vi "example_cmd.vi"() -> ()   [LabVIEW 2015]
uses:
  dotnet_system_exec/dotnet_system_exec.lvclass
panel:
  in  "working directory":path=path "c:/"
  out "StdErr":string
  out "StdOut":string
  in  "Send":bool
  in  "Cmd In (can include multiple lines)":string="dir"
  in  "Stop":bool
  # "This examples launches the cmd.exe process and allows you to send strings via stdin, while asynchronously listening to stdout and stderr  \n\nCalling \"exit\" in CmdIn will stop the cmd.exe instance and stop this VI. You can leverage this by adding a final exit line after the command(s)\nyou wish to send to have this VI auto-terminate upon completion."
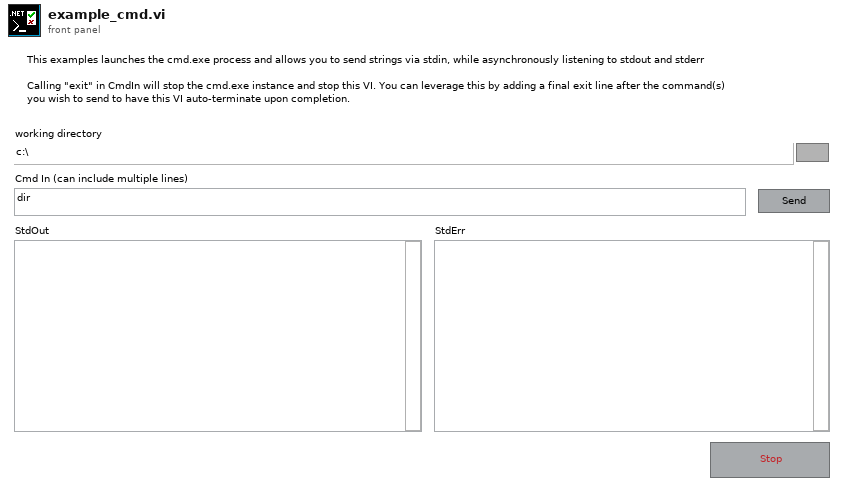
[diagram p1: front panel]
types:
  T1 = cluster{"stdout event":refnum<user-event>, "stderr event":refnum<user-event>, "process_exit event":refnum<user-event>}
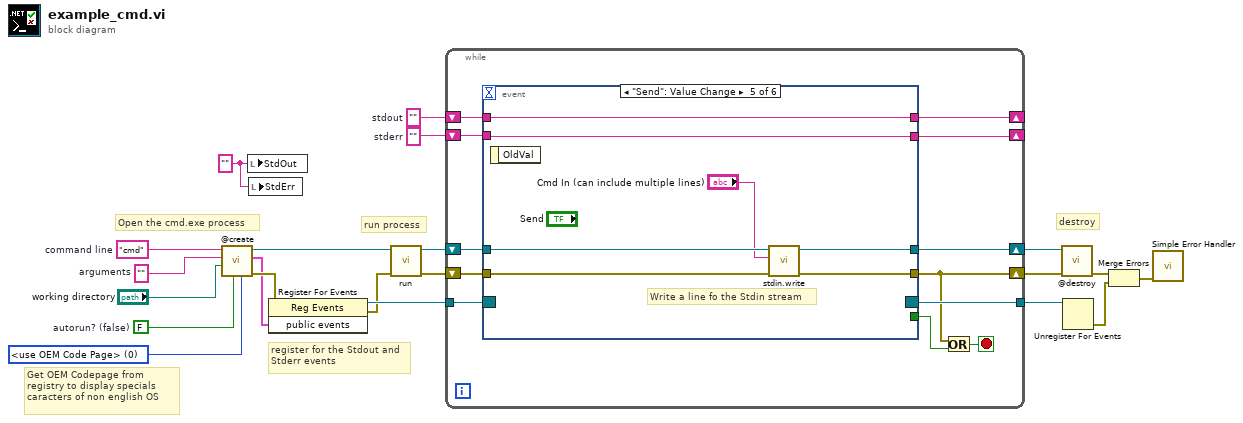
[diagram p0: block diagram]
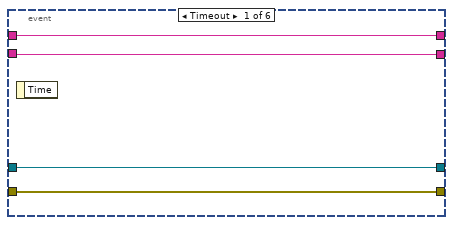
[diagram p2: hidden frame]
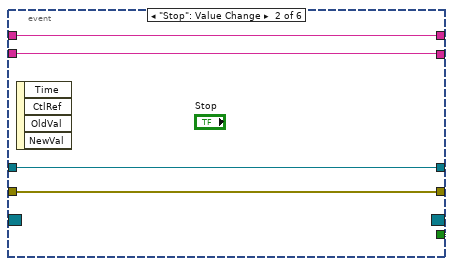
[diagram p3: hidden frame]
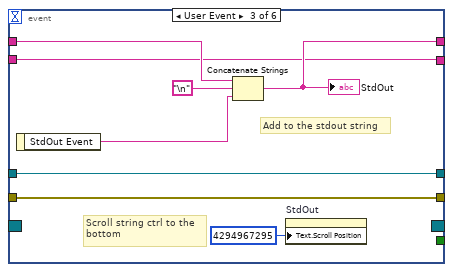
[diagram p4: hidden frame]
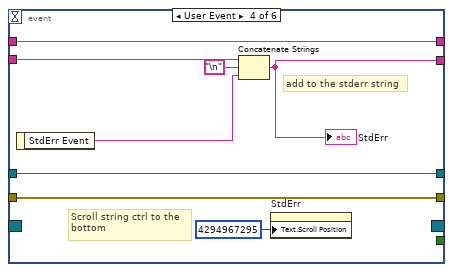
[diagram p5: hidden frame]
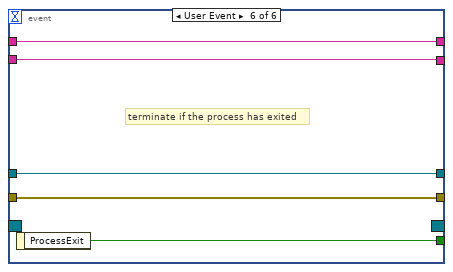
[diagram p6: hidden frame]
diagram:
  w1 = 0 items=["<do not specify>"=-1, "<use OEM Code Page>"=0, "IBM037 - IBM EBCDIC US-Canada"=37, "IBM437 - OEM United States"=437, "IBM500 - IBM EBCDIC International"=500, "ASMO-708 - Arabic (ASMO 708)"=708, "709 - Arabic (ASMO-449+, BCON V4)"=709, "710 - Arabic - Transparent Arabic"=710, "DOS-720 - Arabic (Transparent ASMO); Arabic (DOS)"=720, "ibm737 - OEM Greek (formerly 437G); Greek (DOS)"=737, "ibm775 - OEM Baltic; Baltic (DOS)"=775, "ibm850 - OEM Multilingual Latin 1; Western European (DOS)"=850, "ibm852 - OEM Latin 2; Central European (DOS)"=852, "IBM855 - OEM Cyrillic (primarily Russian)"=855, "ibm857 - OEM Turkish; Turkish (DOS)"=857, "IBM00858 - OEM Multilingual Latin 1 + Euro symbol"=858, "IBM860 - OEM Portuguese; Portuguese (DOS)"=860, "ibm861 - OEM Icelandic; Icelandic (DOS)"=861, "DOS-862 - OEM Hebrew; Hebrew (DOS)"=862, "IBM863 - OEM French Canadian; French Canadian (DOS)"=863, "IBM864 - OEM Arabic; Arabic (864)"=864, "IBM865 - OEM Nordic; Nordic (DOS)"=865, "cp866 - OEM Russian; Cyrillic (DOS)"=866, "ibm869 - OEM Modern Greek; Greek, Modern (DOS)"=869, "IBM870 - IBM EBCDIC Multilingual/ROECE (Latin 2); IBM EBCDIC Multilingual Latin 2"=870, "windows-874 - Thai (Windows)"=874, "cp875 - IBM EBCDIC Greek Modern"=875, "shift_jis - ANSI/OEM Japanese; Japanese (Shift-JIS)"=932, "gb2312 - ANSI/OEM Simplified Chinese (PRC, Singapore); Chinese Simplified (GB2312)"=936, "ks_c_5601-1987 - ANSI/OEM Korean (Unified Hangul Code)"=949, "big5 - ANSI/OEM Traditional Chinese (Taiwan; Hong Kong SAR, PRC); Chinese Traditional (Big5)"=950, "IBM1026 - IBM EBCDIC Turkish (Latin 5)"=1026, "IBM01047 - IBM EBCDIC Latin 1/Open System"=1047, "IBM01140 - IBM EBCDIC US-Canada (037 + Euro symbol); IBM EBCDIC (US-Canada-Euro)"=1140, "IBM01141 - IBM EBCDIC Germany (20273 + Euro symbol); IBM EBCDIC (Germany-Euro)"=1141, "IBM01142 - IBM EBCDIC Denmark-Norway (20277 + Euro symbol); IBM EBCDIC (Denmark-Norway-Euro)"=1142, "IBM01143 - IBM EBCDIC Finland-Sweden (20278 + Euro symbol); IBM EBCDIC (Finland-Sweden-Euro)"=1143, "IBM01144 - IBM EBCDIC Italy (20280 + Euro symbol); IBM EBCDIC (Italy-Euro)"=1144, "IBM01145 - IBM EBCDIC Latin America-Spain (20284 + Euro symbol); IBM EBCDIC (Spain-Euro)"=1145, "IBM01146 - IBM EBCDIC United Kingdom (20285 + Euro symbol); IBM EBCDIC (UK-Euro)"=1146, "IBM01147 - IBM EBCDIC France (20297 + Euro symbol); IBM EBCDIC (France-Euro)"=1147, "IBM01148 - IBM EBCDIC International (500 + Euro symbol); IBM EBCDIC (International-Euro)"=1148, "IBM01149 - IBM EBCDIC Icelandic (20871 + Euro symbol); IBM EBCDIC (Icelandic-Euro)"=1149, "utf-16 - Unicode UTF-16, little endian byte order (BMP of ISO 10646); available only to managed applications"=1200, "unicodeFFFE - Unicode UTF-16, big endian byte order; available only to managed applications"=1201, "windows-1250 - ANSI Central European; Central European (Windows)"=1250, "windows-1251 - ANSI Cyrillic; Cyrillic (Windows)"=1251, "windows-1252 - ANSI Latin 1; Western European (Windows)"=1252, "windows-1253 - ANSI Greek; Greek (Windows)"=1253, "windows-1254 - ANSI Turkish; Turkish (Windows)"=1254, "windows-1255 - ANSI Hebrew; Hebrew (Windows)"=1255, "windows-1256 - ANSI Arabic; Arabic (Windows)"=1256, "windows-1257 - ANSI Baltic; Baltic (Windows)"=1257, "windows-1258 - ANSI/OEM Vietnamese; Vietnamese (Windows)"=1258, "Johab - Korean (Johab)"=1361, "macintosh - MAC Roman; Western European (Mac)"=10000, "x-mac-japanese - Japanese (Mac)"=10001, "x-mac-chinesetrad - MAC Traditional Chinese (Big5); Chinese Traditional (Mac)"=10002, "x-mac-korean - Korean (Mac)"=10003, "x-mac-arabic - Arabic (Mac)"=10004, "x-mac-hebrew - Hebrew (Mac)"=10005, "x-mac-greek - Greek (Mac)"=10006, "x-mac-cyrillic - Cyrillic (Mac)"=10007, "x-mac-chinesesimp - MAC Simplified Chinese (GB 2312); Chinese Simplified (Mac)"=10008, "x-mac-romanian - Romanian (Mac)"=10010, "x-mac-ukrainian - Ukrainian (Mac)"=10017, "x-mac-thai - Thai (Mac)"=10021, "x-mac-ce - MAC Latin 2; Central European (Mac)"=10029, "x-mac-icelandic - Icelandic (Mac)"=10079, "x-mac-turkish - Turkish (Mac)"=10081, "x-mac-croatian - Croatian (Mac)"=10082, "utf-32 - Unicode UTF-32, little endian byte order; available only to managed applications"=12000, "utf-32BE - Unicode UTF-32, big endian byte order; available only to managed applications"=12001, "x-Chinese_CNS - CNS Taiwan; Chinese Traditional (CNS)"=20000, "x-cp20001 - TCA Taiwan"=20001, "x_Chinese-Eten - Eten Taiwan; Chinese Traditional (Eten)"=20002, "x-cp20003 - IBM5550 Taiwan"=20003, "x-cp20004 - TeleText Taiwan"=20004, "x-cp20005 - Wang Taiwan"=20005, "x-IA5 - IA5 (IRV International Alphabet No. 5, 7-bit); Western European (IA5)"=20105, "x-IA5-German - IA5 German (7-bit)"=20106, "x-IA5-Swedish - IA5 Swedish (7-bit)"=20107, "x-IA5-Norwegian - IA5 Norwegian (7-bit)"=20108, "us-ascii - US-ASCII (7-bit)"=20127, "x-cp20261 - T.61"=20261, "x-cp20269 - ISO 6937 Non-Spacing Accent"=20269, "IBM273 - IBM EBCDIC Germany"=20273, "IBM277 - IBM EBCDIC Denmark-Norway"=20277, "IBM278 - IBM EBCDIC Finland-Sweden"=20278, "IBM280 - IBM EBCDIC Italy"=20280, "IBM284 - IBM EBCDIC Latin America-Spain"=20284, "IBM285 - IBM EBCDIC United Kingdom"=20285, "IBM290 - IBM EBCDIC Japanese Katakana Extended"=20290, "IBM297 - IBM EBCDIC France"=20297, "IBM420 - IBM EBCDIC Arabic"=20420, "IBM423 - IBM EBCDIC Greek"=20423, "IBM424 - IBM EBCDIC Hebrew"=20424, "x-EBCDIC-KoreanExtended - IBM EBCDIC Korean Extended"=20833, "IBM-Thai - IBM EBCDIC Thai"=20838, "koi8-r - Russian (KOI8-R); Cyrillic (KOI8-R)"=20866, "IBM871 - IBM EBCDIC Icelandic"=20871, "IBM880 - IBM EBCDIC Cyrillic Russian"=20880, "IBM905 - IBM EBCDIC Turkish"=20905, "IBM00924 - IBM EBCDIC Latin 1/Open System (1047 + Euro symbol)"=20924, "EUC-JP - Japanese (JIS 0208-1990 and 0212-1990)"=20932, "x-cp20936 - Simplified Chinese (GB2312); Chinese Simplified (GB2312-80)"=20936, "x-cp20949 - Korean Wansung"=20949, "cp1025 - IBM EBCDIC Cyrillic Serbian-Bulgarian"=21025, "21027 - (deprecated)"=21027, "koi8-u - Ukrainian (KOI8-U); Cyrillic (KOI8-U)"=21866, "iso-8859-1 - ISO 8859-1 Latin 1; Western European (ISO)"=28591, "iso-8859-2 - ISO 8859-2 Central European; Central European (ISO)"=28592, "iso-8859-3 - ISO 8859-3 Latin 3"=28593, "iso-8859-4 - ISO 8859-4 Baltic"=28594, "iso-8859-5 - ISO 8859-5 Cyrillic"=28595, "iso-8859-6 - ISO 8859-6 Arabic"=28596, "iso-8859-7 - ISO 8859-7 Greek"=28597, "iso-8859-8 - ISO 8859-8 Hebrew; Hebrew (ISO-Visual)"=28598, "iso-8859-9 - ISO 8859-9 Turkish"=28599, "iso-8859-13 - ISO 8859-13 Estonian"=28603, "iso-8859-15 - ISO 8859-15 Latin 9"=28605, "x-Europa - Europa 3"=29001, "iso-8859-8-i - ISO 8859-8 Hebrew; Hebrew (ISO-Logical)"=38598, "iso-2022-jp - ISO 2022 Japanese with no halfwidth Katakana; Japanese (JIS)"=50220, "csISO2022JP - ISO 2022 Japanese with halfwidth Katakana; Japanese (JIS-Allow 1 byte Kana)"=50221, "iso-2022-jp - ISO 2022 Japanese JIS X 0201-1989; Japanese (JIS-Allow 1 byte Kana - SO/SI)"=50222, "iso-2022-kr - ISO 2022 Korean"=50225, "x-cp50227 - ISO 2022 Simplified Chinese; Chinese Simplified (ISO 2022)"=50227, "50229 - ISO 2022 Traditional Chinese"=50229, "50930 - EBCDIC Japanese (Katakana) Extended"=50930, "50931 - EBCDIC US-Canada and Japanese"=50931, "50933 - EBCDIC Korean Extended and Korean"=50933, "50935 - EBCDIC Simplified Chinese Extended and Simplified Chinese"=50935, "50936 - EBCDIC Simplified Chinese"=50936, "50937 - EBCDIC US-Canada and Traditional Chinese"=50937, "50939 - EBCDIC Japanese (Latin) Extended and Japanese"=50939, "euc-jp - EUC Japanese"=51932, "EUC-CN - EUC Simplified Chinese; Chinese Simplified (EUC)"=51936, "euc-kr - EUC Korean"=51949, "51950 - EUC Traditional Chinese"=51950, "hz-gb-2312 - HZ-GB2312 Simplified Chinese; Chinese Simplified (HZ)"=52936, "GB18030 - Windows XP and later: GB18030 Simplified Chinese (4 byte); Chinese Simplified (GB18030)"=54936, "x-iscii-de - ISCII Devanagari"=57002, "x-iscii-be - ISCII Bangla"=57003, "x-iscii-ta - ISCII Tamil"=57004, "x-iscii-te - ISCII Telugu"=57005, "x-iscii-as - ISCII Assamese"=57006, "x-iscii-or - ISCII Odia"=57007, "x-iscii-ka - ISCII Kannada"=57008, "x-iscii-ma - ISCII Malayalam"=57009, "x-iscii-gu - ISCII Gujarati"=57010, "x-iscii-pa - ISCII Punjabi"=57011, "utf-7 - Unicode (UTF-7)"=65000, "utf-8 - Unicode (UTF-8)"=65001] ("CodePage (<do not specify>)")
  w2 = FALSE  # autorun? (false)
  w3 = "" ("Process File Name")
  w5 = ""  # stderr
  w10 = ""  # arguments
  w11 = ""  # stdout
  w12 = "cmd"  # command line
  # "Get OEM Codepage from registry to display specials caracters of non english OS"
  # "destroy"
  # "register for the Stdout and\nStderr events"
  # "run process"
  # "Open the cmd.exe process"
  n1 = call "@create.vi"("CodePage (<do not specify>)"=w1, "autorun? (false)"=w2, "working directory (c:\\)"="working directory", "arguments (\"\")"=w10, "command line (cmd.exe)"=w12) -> ("error out"=w8:errorcluster, "public events"=w6:T1, "dotnet_system_exec out"=w19:refnum<class "dotnet_system_exec.lvclass">)  [unwired: 4 in]
  n2 = local write "StdOut"(w3) -> ()
  n3 = local write "StdErr"(w3) -> ()
  n4 = register-events(error in=w8, w6) -> (reference out=w18:refnum<event-registration>, error out=w7:errorcluster)  [unwired: 1 in]
  n5 = call "run.vi"("error in (no error)"=w7, "dotnet_system_exec in"=w19) -> ("error out"=w9:errorcluster, "dotnet_system_exec out"=w21:refnum<class "dotnet_system_exec.lvclass">)  [unwired: 8 in]
  n6 = while {
    shift-right: [w33] -> w20
    shift-left: w21 -> [w32]
    shift-right: [w23] -> w16
    shift-left: w9 -> [w31]
    tunnel: w18 -> [w30]
    tunnel: [w29] -> w17
    shift-right: [w27] -> _
    shift-left: w11 -> [w28]
    shift-right: [w25] -> _
    shift-left: w5 -> [w26]
    stop <- w22 stop-if-true
    n7 = event shown="[4] \"Send\": Value Change" {
      selector: w30 -> [_ _ _ _ _ _]
      dyn-events: [_ _ _ _ _ _] -> w29
      timeout: _ -> [_ _ _ _ _ _]
      tunnel: [w37 w42 w50 w58 w65 w67] -> w33
      tunnel: w32 -> [w37 w42 w50 w58 w64 w67]
      tunnel: w31 -> [w36 w41 w49 w57 w62 w66]
      tunnel: [w36 w41 w49 w57 w63 w66] -> w23
      tunnel: w28 -> [w35 w39 w46 w53 w60 w68]
      tunnel: [w35 w39 w47 w53 w60 w68] -> w27
      tunnel: [_ TRUE _ _ _ w70] -> w24
      tunnel: w26 -> [w34 w38 w44 w54 w59 w69]
      tunnel: [w34 w38 w44 w52 w59 w69] -> w25
      event Timeout {
        n8 = event-data() -> ()  [unwired: 1 in, 1 out]
      }
      event "Stop": Value Change {
        n9 = event-data() -> ()  [unwired: 1 in, 4 out]
      }
      event User Event {
        # "Scroll string ctrl to the \nbottom"
        # "Add to the stdout string"
        n10 = event-data() -> ("StdOut Event"=w45:string)  [unwired: 1 in]
        n11 = Concatenate Strings(w46, "\n", w45) -> (w47:string)
        "StdOut" <- w47
        n12 = property on="StdOut" class="Str"("Text.Scroll Position"=u32 4294967295) -> ()  [unwired: 2 in, 2 out]
      }
      event User Event {
        # "Scroll string ctrl to the \nbottom"
        # "add to the stderr string"
        n13 = event-data() -> ("StdErr Event"=w55:string)  [unwired: 1 in]
        n14 = Concatenate Strings(w54, "\n", w55) -> (w52:string)
        "StdErr" <- w52
        n15 = property on="StdErr" class="Str"("Text.Scroll Position"=u32 4294967295) -> ()  [unwired: 2 in, 2 out]
      }
      event "Send": Value Change {
        # "Write a line fo the Stdin stream"
        n16 = event-data() -> ()  [unwired: 1 in, 1 out]
        n17 = call-dynamic "stdin.write.vi"("error in (no error)"=w62, "stdin"="Cmd In (can include multiple lines)", "dotnet_system_exec in"=w64) -> ("error out"=w63:errorcluster, "dotnet_system_exec out"=w65:refnum<class "dotnet_system_exec.lvclass">)  [unwired: 7 in]
      }
      event User Event {
        # "terminate if the process has exited"
        n18 = event-data() -> ("ProcessExit"=w70:bool)  [unwired: 1 in]
      }
    }
    n19 = Or(x=w23, y=w24) -> (x .or. y?=w22:bool)
  }
  n20 = call-dynamic "@destroy.vi"("error in (no error)"=w16, "dotnet_system_exec in"=w20) -> ("error out"=w15:errorcluster)  [unwired: 8 in, 1 out]
  n21 = Unregister For Events(event registration refnum=w17) -> (error out=w14:errorcluster)  [unwired: 1 in]
  n22 = Merge Errors(w15, w14) -> (w13:errorcluster)
  n23 = call <vilib>:"Simple Error Handler.vi"("error in (no error)"=w13) -> ()  [unwired: 4 in, 5 out]
